vi "Reset ROI.vi"(11 "Section Graph. in":refnum<class "Graph with Section Views.lvclass">) -> (3 "Section Graph. out":refnum<class "Graph with Section Views.lvclass">)   [LabVIEW 2023, in "Graph with Section Views.lvclass"]
uses:
  Graph with Section Views.lvclass
  Graph with Section Views.lvclass/Graph with Section Views.ctl
  Base Graph/Base Graph.lvclass
  D:/git/Lock-In-Thermography-Graphs/source/Base Graph/Base Graph.lvclass
  D:/git/Lock-In-Thermography-Graphs/source/Detail Graph/Graph with Section Views.lvclass
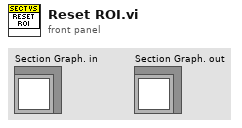
[diagram p1: front panel]
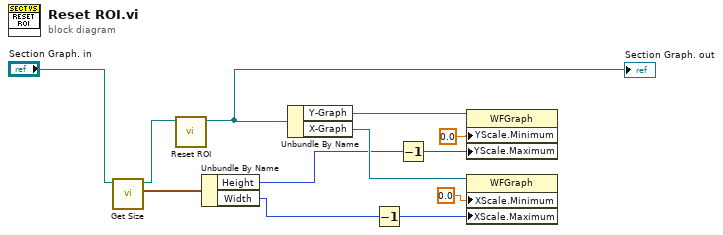
[diagram p0: block diagram]
diagram:
  n1 = call "Get Size.vi"("TG Base Graph in"="Section Graph. in") -> ("Sizes"=w5:cluster{"Height":u32, "Width":u32}, "TG Base Graph out"=w6:refnum<class "Graph with Section Views.lvclass">)  [unwired: 9 in]
  n2 = call-parent "Reset ROI.vi"("TG Base Graph in"=w6) -> ("TG Base Graph out"=w12:refnum<class "Graph with Section Views.lvclass">)  [unwired: 10 in]
  "Section Graph. out" <- w12
  n3 = Unbundle By Name(w5) -> ("Height"=w4:u32, "Width"=w2:u32)
  n4 = Unbundle By Name(w12) -> ("Y-Graph"=w10:refnum<vi>, "X-Graph"=w9:refnum<vi>)
  n5 = Decrement(x=w2) -> (x-1=w1:u32)
  n6 = Decrement(x=w4) -> (x-1=w3:u32)
  n7 = property class="WFGraph"(reference=w10, "YScale.Minimum"=0.0 ("Y Scale.Range:Minimum"), "YScale.Maximum"=w3) -> ()  [unwired: 1 in, 2 out]
  n8 = property class="WFGraph"(reference=w9, "XScale.Minimum"=0.0 ("X Scale.Range:Minimum"), "XScale.Maximum"=w1) -> ()  [unwired: 1 in, 2 out]
